vi "Test Info.vi"(8 "error in (no error)":errorcluster, 10 "Test info":T1, 11 "MySQL in":refnum<class "MySQL.lvclass">) -> (0 "error out":errorcluster, 3 "MySQL out":refnum<class "MySQL.lvclass">)   [LabVIEW 2021, in "Database.lvlib" / "MySQL.lvclass"]
uses:
  MySQL.lvclass
  MySQL.lvclass/MySQL.ctl
  <vilib>/addons/database/NI_Database_API.lvlib
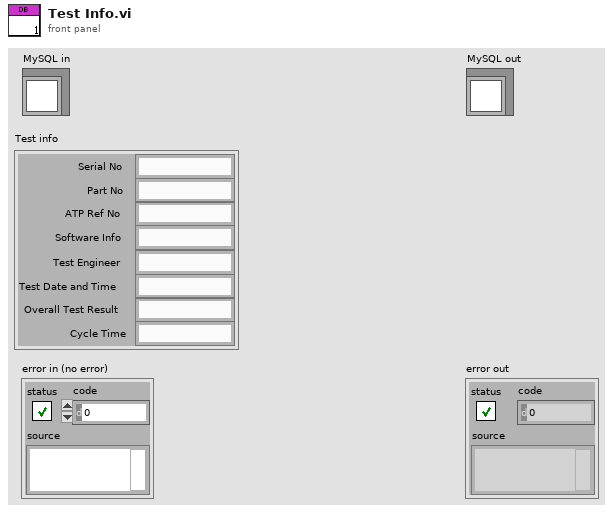
[diagram p1: front panel]
types:
  T1 = cluster{"Serial No":string, "Part No":string, "ATP Ref No":string, "Software Info":string, "Test Engineer":string, "Test Date and Time":string, "Overall Test Result":string, "Cycle Time":string}
  T2 = typedef "Database.lvlib/DB.lvclass/Table_info.ctl" = cluster{"Authentication":string, "Instr_Configuration":string, "Recipe":string, "Test_data":string}
  T3 = typedef "NI_Database_API.lvlib/Conn ObjectReference.ctl" = refnum<k1>
  T4 = cluster{"[0]":string, "[1]":string, "[2]":string, "[3]":string, "[4]":string, "[5]":string, "[6]":string, "[7]":string, "[8]":string, "[9]":string, "[10]":string, "[11]":string, "[12]":string, "[13]":string}
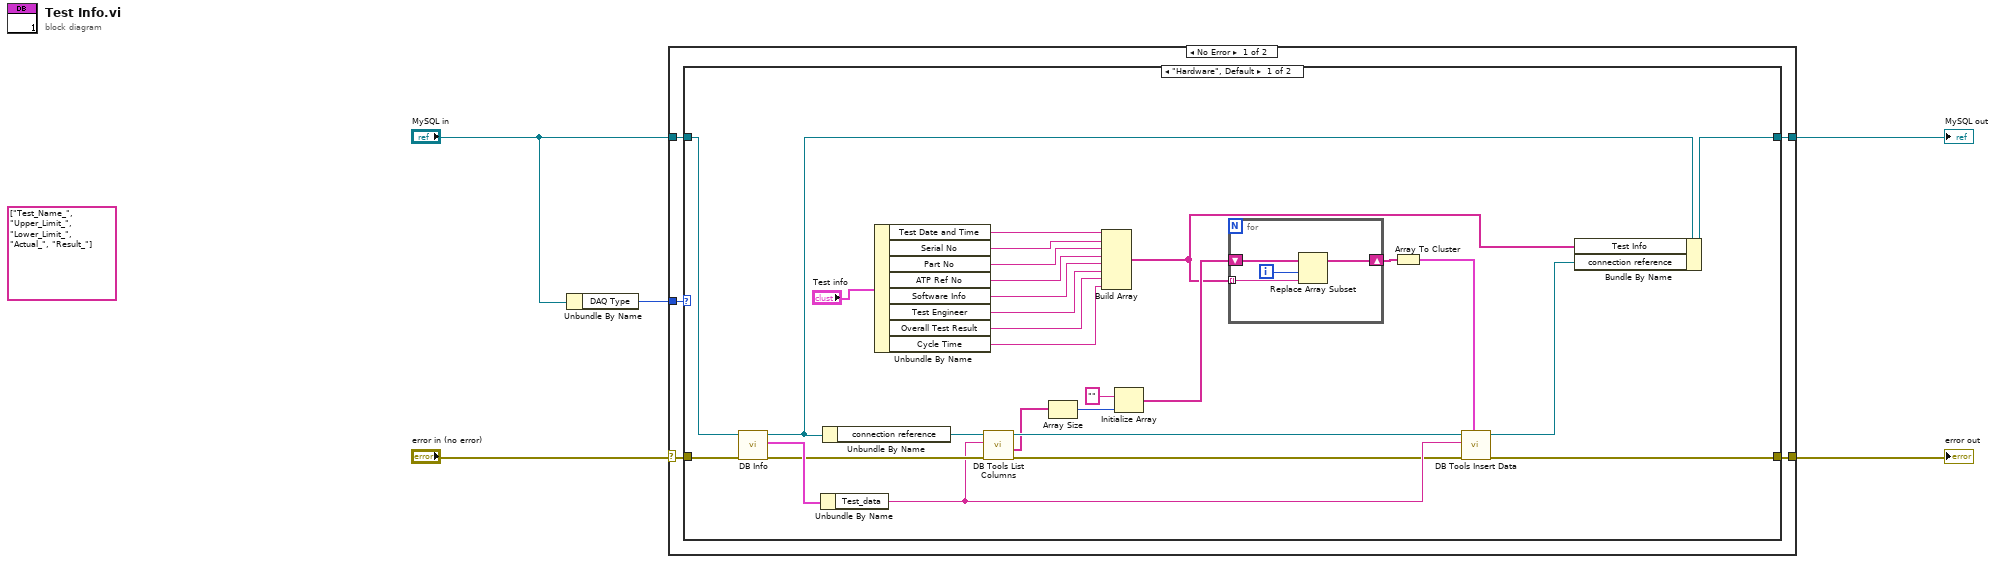
[diagram p0: block diagram]
diagram:
  (unwired) string[] ["Test_Name_", "Upper_Limit_", "Lower_Limit_", "Actual_", "Result_"]
  n1 = Unbundle By Name("MySQL in") -> ("DAQ Type"=w3:enum16{"Hardware", "Simulation"})
  n2 = case shown="No Error" "error in (no error)" {
    selector: "error in (no error)" -> [w7 w45]
    tunnel: "MySQL in" -> [w9 w46]
    tunnel: w3 -> [w10 _]
    tunnel: [w8 w46] -> w2
    tunnel: [w6 w45] -> w1
    frame No Error {
      n3 = case shown="\"Hardware\", Default" w10 {
        tunnel: w9 -> [w38 w44]
        tunnel: [w35 w44] -> w8
        tunnel: w7 -> [w37 w43]
        tunnel: [w33 w43] -> w6
        frame "Hardware", Default {
          n4 = call-dynamic "DB Info.vi"("error in (no error)"=w37, "MySQL in"=w38) -> ("error out"=w32:errorcluster, "Table_info"=w36:T2, "MySQL out"=w31:refnum<class "MySQL.lvclass">)  [unwired: 6 in, 1 out]
          n5 = Unbundle By Name(w36) -> ("Test_data"=w29:string)
          n6 = Unbundle By Name(w31) -> ("connection reference"=w30:T3)
          n7 = Unbundle By Name("Test info") -> ("Test Date and Time"=w15:string, "Serial No"=w20:string, "Part No"=w19:string, "ATP Ref No"=w18:string, "Software Info"=w17:string, "Test Engineer"=w16:string, "Overall Test Result"=w14:string, "Cycle Time"=w13:string)
          n8 = call <vilib>:"DB Tools List Columns.vi"("error in (no error)"=w32, "table"=w29, "connection reference"=w30) -> ("error out"=w28:errorcluster, "columns"=w26:string[], "connection reference out"=w27:T3)  [unwired: 1 in, 1 out]
          n9 = Array Size(array=w26) -> (size(s)=w25:i32)
          n10 = Build Array(w15, w20, w19, w18, w17, w16, w14, w13) -> (w12:string[])
          n11 = Initialize Array("", w25) -> (w22:string[])
          n12 = for {
            tunnel: w12 -> [w41] mode=indexing
            shift-right: [w40] -> w21
            shift-left: w22 -> [w39]
            i -> [w42]
            n13 = Replace Array Subset(array=w39, new element=w41, index=w42) -> (w40:string[])
          }
          n14 = Array To Cluster(array=w21) -> (cluster=w23:T4)
          n15 = call <vilib>:"DB Tools Insert Data.vi"("data"=w23, "error in (no error)"=w28, "table"=w29, "connection reference"=w27) -> ("error out"=w33:errorcluster, "connection reference out"=w34:T3)  [unwired: 6 in]
          n16 = Bundle By Name(cluster=w31, "Test Info"=w12, "connection reference"=w34) -> (w35:refnum<class "MySQL.lvclass">)
        }
        frame "Simulation" {
        }
      }
    }
    frame Error {
    }
  }
  "error out" <- w1
  "MySQL out" <- w2
